vi "In Limits Status.vi"(7 "Channel (0: Channel A)":u16(ring) items=["Channel A", "Channel B"], 8 "error in (no error)":errorcluster, 11 "BH Druck PACE Series in":refnum<class "BH Druck PACE Series.lvclass">) -> (0 "error out":errorcluster, 1 "Time to In Limits /s":dbl, 2 "In Limits":bool, 3 "BH Druck PACE Series out":refnum<class "BH Druck PACE Series.lvclass">, 4 "Time to In Limits":string)   [LabVIEW 2022 SP3, in "BH Druck PACE Series.lvclass"]
uses:
  BH Druck PACE Series.lvclass
  BH Druck PACE Series.lvclass/BH Druck PACE Series.ctl
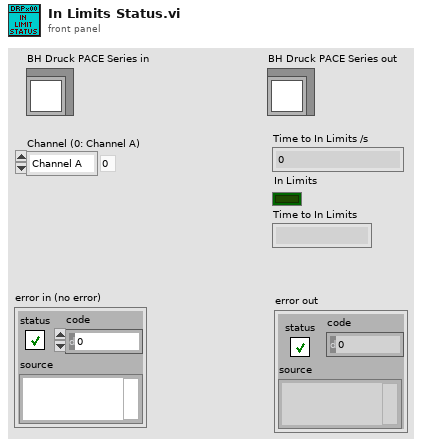
[diagram p1: front panel]
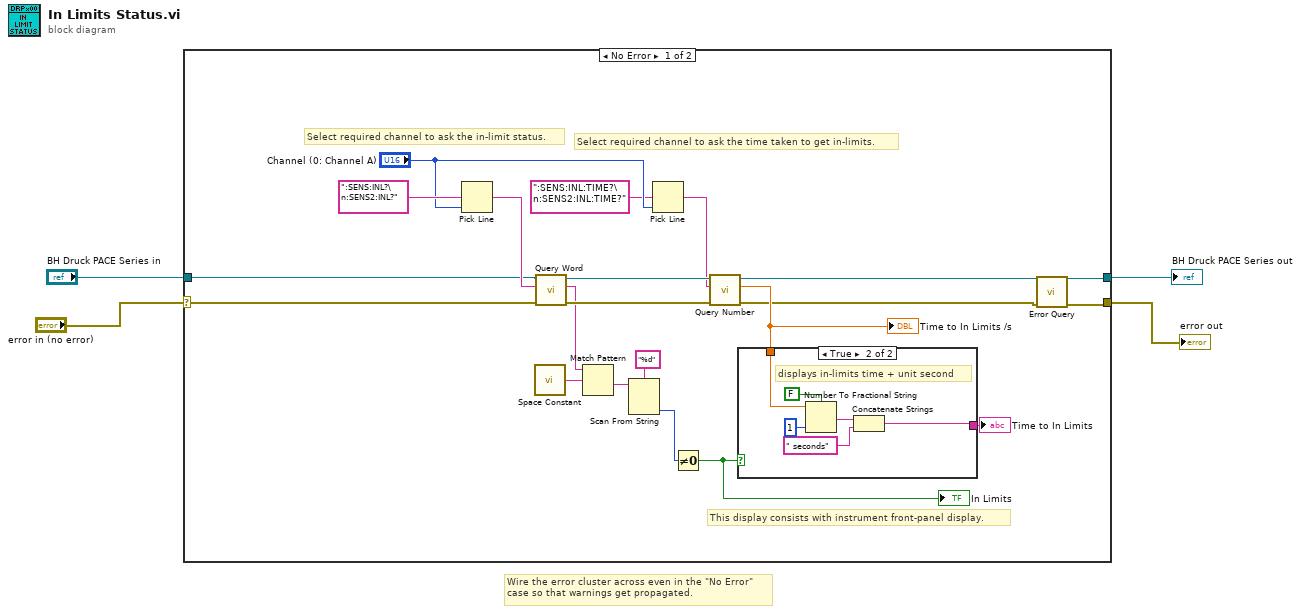
[diagram p0: block diagram]
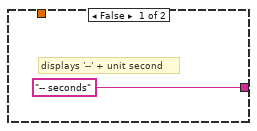
[diagram p2: hidden frame]
diagram:
  # "Wire the error cluster across even in the \"No Error\"\ncase so that warnings get propagated."
  n1 = case shown="No Error" "error in (no error)" {
    selector: "error in (no error)" -> [w10 w34]
    tunnel: [w5 w34] -> w3
    tunnel: [w6 w33] -> w1
    tunnel: "BH Druck PACE Series in" -> [w9 w33]
    frame No Error {
      # "Select required channel to ask the time taken to get in-limits."
      # "Select required channel to ask the in-limit status."
      # "This display consists with instrument front-panel display."
      n2 = Pick Line(multi-line string=":SENS:INL?\n:SENS2:INL?", line index="Channel (0: Channel A)") -> (output string=w14:string)  [unwired: 1 in]
      n3 = call <vilib>:"Space Constant.vi"() -> ("String"=w22:string)
      n4 = call-dynamic "Query Word.vi"("error in (no error)"=w10, "Query String"=w14, "BH Druck PACE Series in"=w9) -> ("error out"=w25:errorcluster, "String Result"=w21:string, "BH Druck PACE Series out"=w24:refnum<class "BH Druck PACE Series.lvclass">)  [unwired: 6 in]
      n5 = Match Pattern(string=w21, regular expression=w22) -> (after substring=w20:string)  [unwired: 1 in, 3 out]
      n6 = Scan From String(format string="%d" ("Format String"), input string=w20) -> (output 1=w19:i32)  [unwired: 3 in, 3 out]
      n7 = Pick Line(multi-line string=":SENS:INL:TIME?\n:SENS2:INL:TIME?", line index="Channel (0: Channel A)") -> (output string=w13:string)  [unwired: 1 in]
      n8 = Not Equal To 0?(x=w19) -> (x != 0?=w16:bool)
      "In Limits" <- w16
      n9 = call-dynamic "Query Number.vi"("error in (no error)"=w25, "Query String"=w13, "BH Druck PACE Series in"=w24) -> ("error out"=w7:errorcluster, "Numeric Result"=w18:dbl, "BH Druck PACE Series out"=w8:refnum<class "BH Druck PACE Series.lvclass">)  [unwired: 6 in]
      "Time to In Limits /s" <- w18
      n10 = case shown="True" w16 {
        tunnel: w18 -> [_ w32]
        tunnel: ["-- seconds" w29] -> w17
        frame False {
          # "displays '--' + unit second"
        }
        frame True {
          # "displays in-limits time + unit second"
          n11 = Number To Fractional String(use system decimal point (T)=FALSE, number=w32, precision (6)=i16 1) -> (F-format string=w30:string)  [unwired: 1 in]
          n12 = Concatenate Strings(w30, " seconds") -> (w29:string)
        }
      }
      "Time to In Limits" <- w17
      n13 = call-dynamic "Error Query.vi"("error in (no error)"=w7, "BH Druck PACE Series in"=w8) -> ("error out"=w5:errorcluster, "BH Druck PACE Series out"=w6:refnum<class "BH Druck PACE Series.lvclass">)  [unwired: 8 in]
    }
    frame Error {
    }
  }
  "error out" <- w3
  "BH Druck PACE Series out" <- w1
